vi "SRV_Sensor Config GUI.vi"(8 "error in (no error)":errorcluster, 9 "Sensor to Edit":string, 11 "Sensors Config File Path in":path) -> (0 "error out":errorcluster, 1 "Cancelled?":bool, 3 "Sensor Config Filepath":path)   [LabVIEW 2009]
doc: "A Producer-Consumer two-loop state machine template. This template uses the LPD Command Queues to drive its execution.\n\nThere are several advantages such as:\n- convenient error state control\n- the ability to pass data between states/loops/VIs via a variant\n- command history which is extremely valuable in troubleshooting when an error occurs\n\n\nAuthor: Mike Schultz\n\nLogicPD, Inc\nwww.logicpd.com"
uses:
  SRV_Sensor Config Cluster.ctl
  SRV_Sensor Analog-Digital.ctl
  SRV_Sensor Sampling Mode.ctl
  SRV_Sensor View Config Cluster.ctl
  SRV_Sensors Names.ctl
  SRV_Sensor PicoC Shared Var Type.ctl
  Support/SRV_Command-Data Queue Data Type.ctl
panel:
  in  "Sensor Config":T1={"Name"="", "A/D"=enum."Analog", "I2C Address"=0, "Register"=0, "Channel"=0, "Digital Mask"=0, "Units"="", "Sampling Mode"=enum."Polled", "Sample Period (ms)"=1000, "Formula"="", "Sensor View Config"={"Sensor Name"=enum."Gauge 01", "Minimum"=0.0, "Maximum"=10.0}, "Active"=FALSE, "PicoC Shared Var Type"=enum."Integer", "Index"=0, "Stream Multiple?"=FALSE, "Index End"=255} caption="Gauge 01" {"Register" format="%.0x"; "I2C Address" format="%.0x"; "Sample Period (ms)" min=10 max=60000 step=1; "Digital Mask" format="%.0x"; "Channel" format="%.0x"}
  in  "Cancel Button":bool
  in  "OK Button":bool
  in  "About":bool
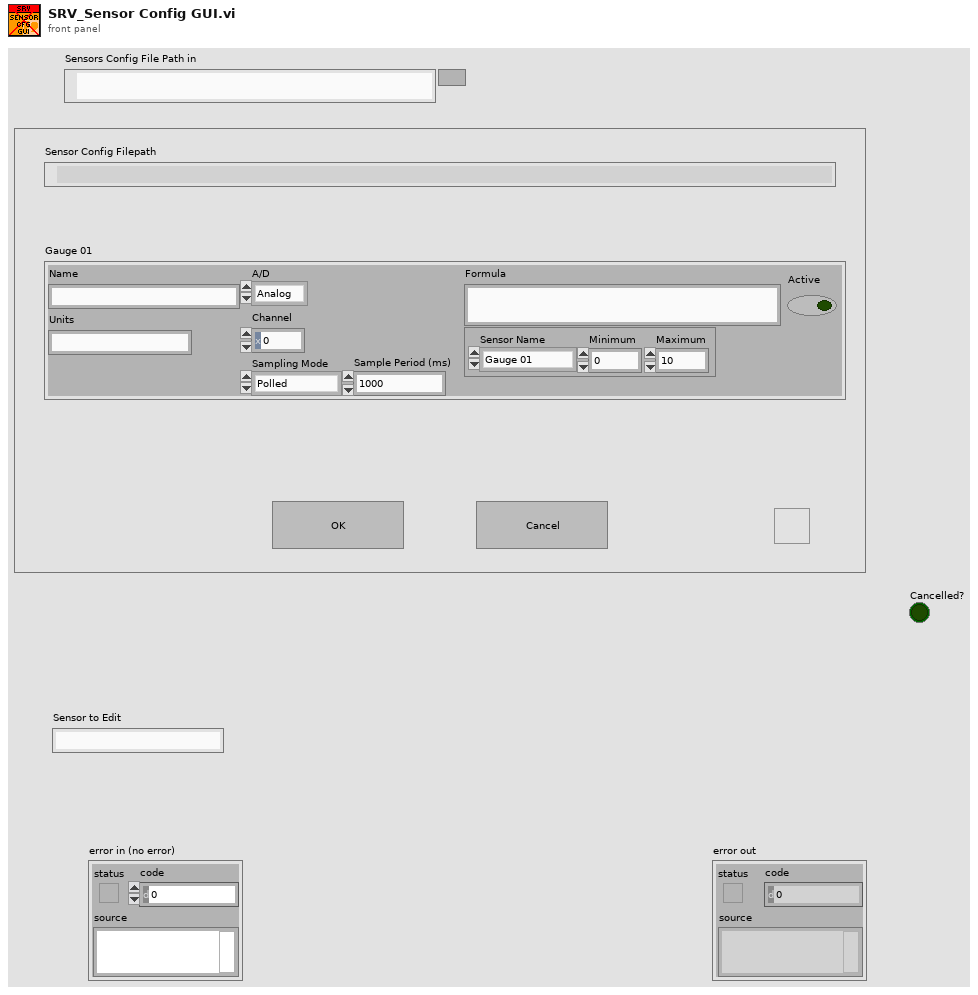
[diagram p1: front panel]
types:
  T1 = typedef "SRV_Sensor Config Cluster.ctl" = cluster{"Name":string, "A/D":T2, "I2C Address":u8, "Register":u8, "Channel":u8, "Digital Mask":u8, "Units":string, "Sampling Mode":T3, "Sample Period (ms)":u32, "Formula":string, "Sensor View Config":T4, "Active":bool, "PicoC Shared Var Type":T6, "Index":u8, "Stream Multiple?":bool, "Index End":u8}
  T2 = typedef "SRV_Sensor Analog-Digital.ctl" = enum16{"Analog", "Digital", "RCMx1 Analog", "PicoC Shared"}
  T3 = typedef "SRV_Sensor Sampling Mode.ctl" = enum16{"Polled", "Streaming"}
  T4 = typedef "SRV_Sensor View Config Cluster.ctl" = cluster{"Sensor Name":T5, "Minimum":dbl, "Maximum":dbl}
  T5 = typedef "SRV_Sensors Names.ctl" = enum16{"Gauge 01", "Gauge 02", "Gauge 03", "Gauge 04", "Meter 01", "Meter 02", "Meter 03", "Meter 04", "Numeric 01", "Numeric 02", "Numeric 03", "Numeric 04", "Numeric 05", "Numeric 06", "Numeric 07", "Numeric 08", "Boolean 01", "Boolean 02", "Boolean 03", "Boolean 04", "Boolean 05", "Boolean 06", "Boolean 07", "Boolean 08", "Boolean 09", "Boolean 10", "Boolean 11", "Boolean 12", "Boolean 13", "Boolean 14", "Boolean 15", "Boolean 16", "Boolean 17", "Boolean 18", "Boolean 19", "Boolean 20", "Boolean 21", "Boolean 22", "Boolean 23", "Boolean 24", "Boolean 25", "Boolean 26", "Boolean 27", "Boolean 28", "Boolean 29", "Boolean 30", "Boolean 31", "Boolean 32"}
  T6 = typedef "SRV_Sensor PicoC Shared Var Type.ctl" = enum16{"String", "Integer", "Float"}
  T7 = typedef "SRV_Command-Data Queue Data Type.ctl" = cluster{"Command":string, "Data":variant}
  T8 = cluster{"user event":refnum<user-event>, "Sensor Config Filepath":path, "Sensors Config":T1[], "Cancelled?":bool, "Sensor to Edit":T5, "Sensor Index":i32}
  T9 = enum8{"Enabled", "Disabled", "Disabled and Grayed Out"}
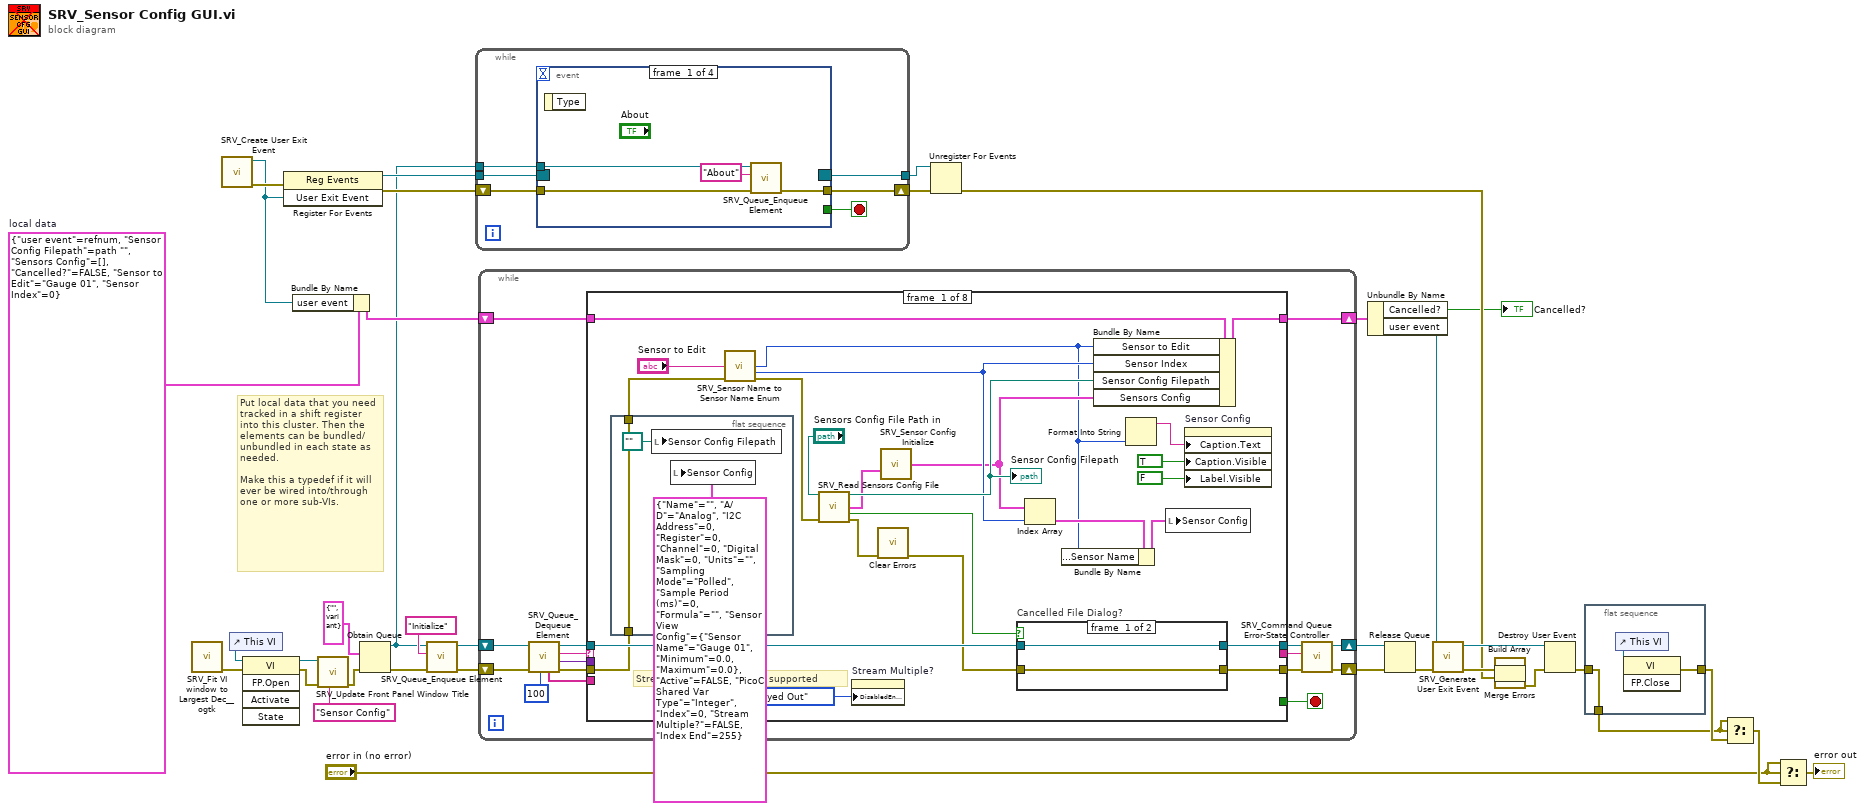
[diagram p0: block diagram]
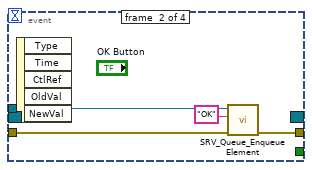
[diagram p2: hidden frame]
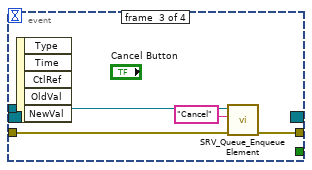
[diagram p3: hidden frame]
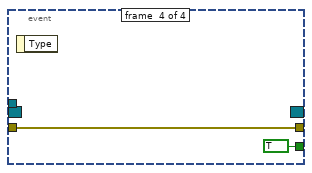
[diagram p4: hidden frame]
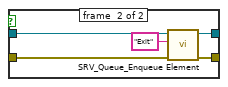
[diagram p5: hidden frame]
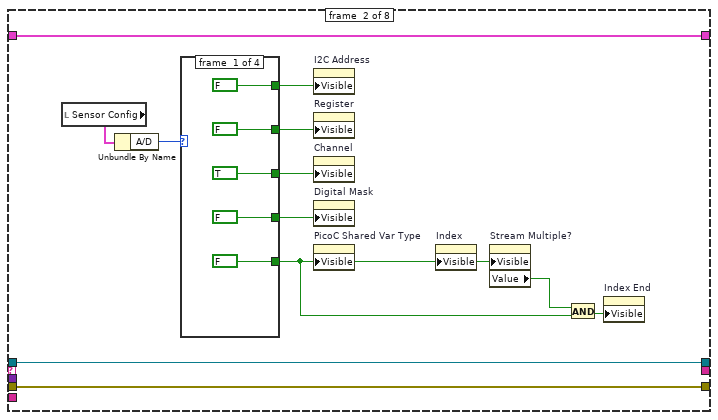
[diagram p6: hidden frame]
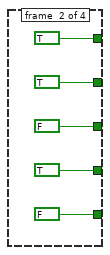
[diagram p7: hidden frame]
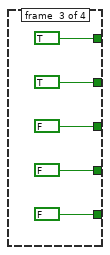
[diagram p8: hidden frame]
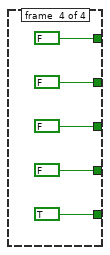
[diagram p9: hidden frame]
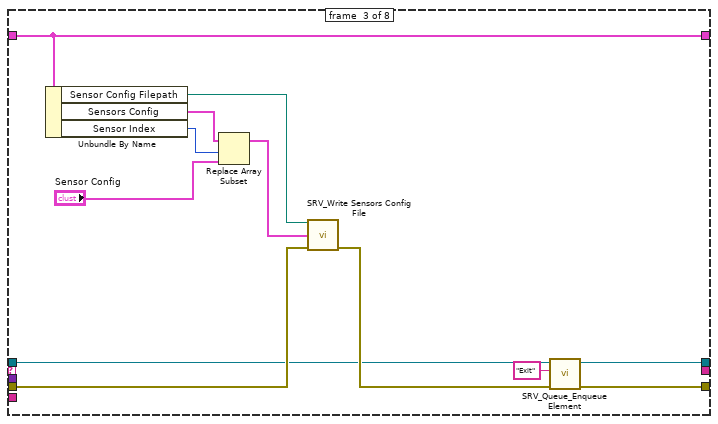
[diagram p10: hidden frame]
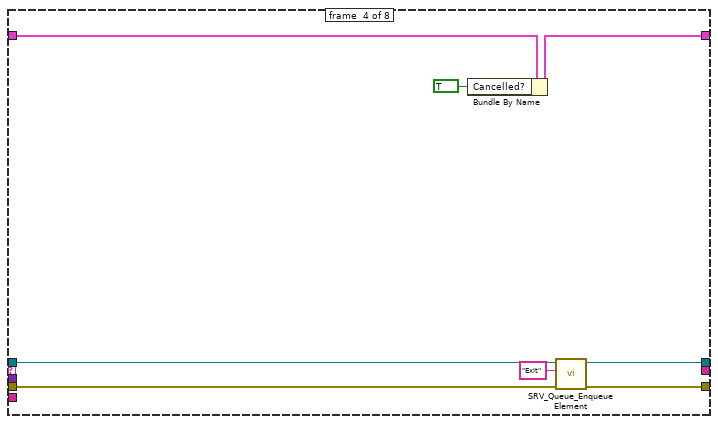
[diagram p11: hidden frame]
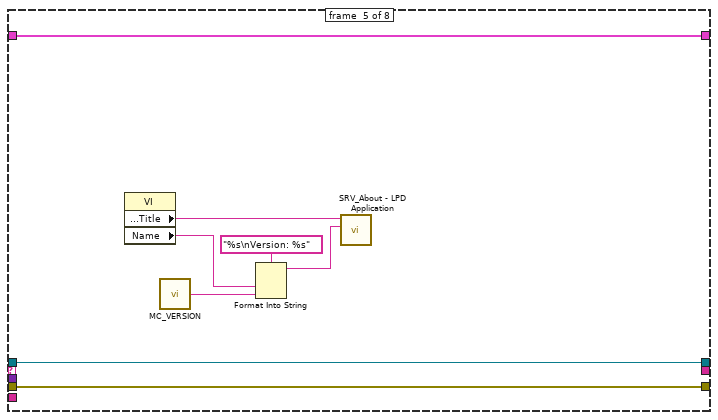
[diagram p12: hidden frame]
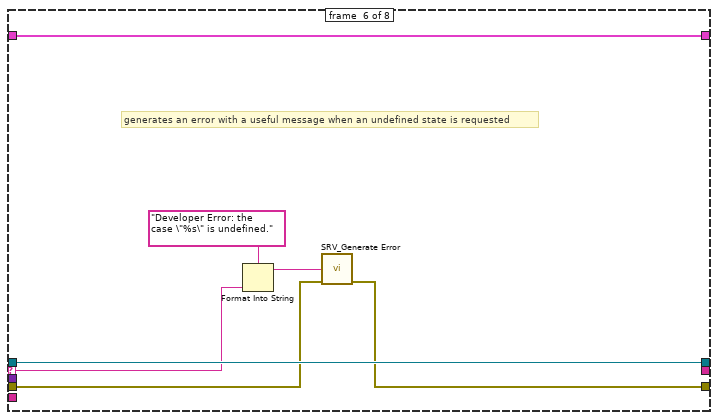
[diagram p13: hidden frame]
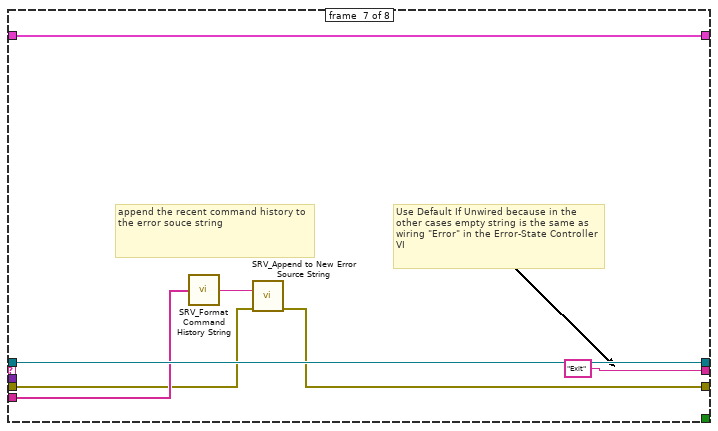
[diagram p14: hidden frame]
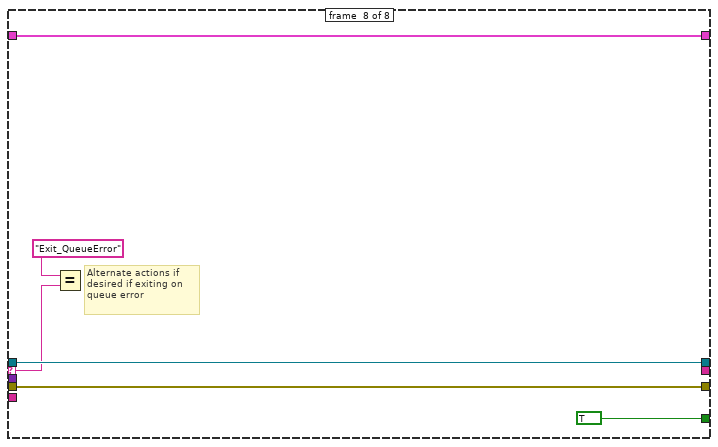
[diagram p15: hidden frame]
diagram:
  w31 = T8 {"user event"=refnum, "Sensor Config Filepath"=path "", "Sensors Config"=[], "Cancelled?"=FALSE, "Sensor to Edit"=enum."Gauge 01", "Sensor Index"=0}  # local data
  # "Put local data that you need tracked in a shift register into this cluster. Then the elements can be bundled/unbundled in each state as needed.\n\nMake this a typedef if it will ever be wired into/through one or more sub-VIs."
  n1 = call "SRV_Fit VI window to Largest Dec__ogtk.vi"() -> ("error out"=w9:errorcluster)  [unwired: 6 in, 1 out]
  n2 = call "SRV_Create User Exit Event.vi"() -> ("error out"=w22:errorcluster, "User Exit Event"=w21:refnum<user-event>)  [unwired: 10 in]
  n3 = control-ref of="This VI"() -> (w10:refnum<vi>)
  n4 = invoke class="VI" method="FP.Open"(reference=w10, error in=w9) -> (reference out=w6:refnum<vi>, error out=w5:errorcluster)  [unwired: 3 in, 3 out]
  n5 = register-events(error in=w22, w21) -> (reference out=w37:refnum<event-registration>, error out=w36:errorcluster)  [unwired: 1 in]
  n6 = Bundle By Name(cluster=w31, "user event"=w21) -> (w30:T8)
  n7 = call "SRV_Update Front Panel Window Title.vi"("Window Title Override String"="Sensor Config", "error in (no error)"=w5, "VI ref"=w6) -> ("error out"=w4:errorcluster)  [unwired: 7 in, 1 out]
  n8 = Obtain Queue(element data type=T7 {"Command"="", "Data"=variant} ("Queue Data Type"), error in (no error)=w4) -> (queue out=w17:refnum<queue>, error out=w18:errorcluster)  [unwired: 3 in, 1 out]
  n9 = call "SRV_Queue_Enqueue Element.vi"("error in (no error)"=w18, "Command"="Initialize", "Command-Data Queue"=w17) -> ("error out"=w14:errorcluster, "Command-Data Queue out"=w16:refnum<queue>)  [unwired: 6 in, 1 out]
  n10 = while {
    shift-right: [w42] -> w34
    shift-left: w36 -> [w43]
    tunnel: w17 -> [w41]
    tunnel: w37 -> [w40]
    tunnel: [w39] -> w35
    stop <- w38 stop-if-true
    n11 = event shown="[2] \"Cancel Button\": Value Change" {
      selector: w40 -> [_ _ _ _]
      dyn-events: [_ _ _ _] -> w39
      timeout: _ -> [_ _ _ _]
      tunnel: w43 -> [w47 w49 w53 w57]
      tunnel: [w46 w50 w54 w57] -> w42
      tunnel: w41 -> [w44 w48 w52 _]
      tunnel: [_ _ _ TRUE] -> w38
      event #0 {
        n12 = event-data() -> ()  [unwired: 1 in, 1 out]
        n13 = call "SRV_Queue_Enqueue Element.vi"("error in (no error)"=w47, "Command"="About", "Command-Data Queue"=w44) -> ("error out"=w46:errorcluster)  [unwired: 6 in, 2 out]
      }
      event #1 {
        n14 = event-data() -> ()  [unwired: 1 in, 5 out]
        n15 = call "SRV_Queue_Enqueue Element.vi"("error in (no error)"=w49, "Command"="OK", "Command-Data Queue"=w48) -> ("error out"=w50:errorcluster)  [unwired: 6 in, 2 out]
      }
      event #2 {
        n16 = event-data() -> ()  [unwired: 1 in, 5 out]
        n17 = call "SRV_Queue_Enqueue Element.vi"("error in (no error)"=w53, "Command"="Cancel", "Command-Data Queue"=w52) -> ("error out"=w54:errorcluster)  [unwired: 6 in, 2 out]
      }
      event #3 {
        n18 = event-data() -> ()  [unwired: 1 in, 1 out]
      }
    }
  }
  n19 = while {
    shift-right: [w67] -> w33
    shift-left: w14 -> [w73]
    shift-right: [w65] -> w32
    shift-left: w16 -> [w71]
    shift-right: [w59] -> w29
    shift-left: w30 -> [w60]
    stop <- w61 stop-if-true
    n20 = call "SRV_Queue_Dequeue Element.vi"("timeout in ms (-1)"=100, "error in (no error)"=w73, "Command-Data Queue"=w71) -> ("error out"=w72:errorcluster, "Data"=w64:variant, "Command"=w69:string, "Command-Data Queue out"=w70:refnum<queue>, "Command History"=w63:string[])  [unwired: 3 in, 1 out]
    n21 = case shown="\"About\"" w69 {
      selector: w69 -> [_ _ _ _ _ w172 _ w184]
      tunnel: w72 -> [w91 w118 w149 w158 w166 w170 w176 w186]
      tunnel: [w95 w118 w146 w157 w166 w169 w177 w186] -> w68
      tunnel: w70 -> [w96 w119 w145 w159 w167 w174 w181 w187]
      tunnel: [w94 w119 w144 w156 w167 w174 w181 w187] -> w66
      tunnel: w64 -> [_ _ _ _ _ _ _ _]
      tunnel: w63 -> [_ _ _ _ _ _ w180 _]
      tunnel: [_ _ _ _ _ _ "Exit" ("Error Command") _] -> w62
      tunnel: [_ _ _ _ _ _ _ TRUE] -> w61
      tunnel: w60 -> [w78 w116 w151 w154 w161 w171 w178 w182]
      tunnel: [w93 w116 w151 w153 w161 w171 w178 w182] -> w59
      frame #0 {
        # "Streaming multiple not yet supported"
        n22 = flat-sequence {
          tunnel: w91 -> [w99]
          tunnel: [w99] -> w88
          frame #0 {
            n23 = local write "Sensor Config Filepath"(path "" ("Sensor Config Filepath")) -> ()
            n24 = local write "Sensor Config"(T1 {"Name"="", "A/D"=enum."Analog", "I2C Address"=0, "Register"=0, "Channel"=0, "Digital Mask"=0, "Units"="", "Sampling Mode"=enum."Polled", "Sample Period (ms)"=0, "Formula"="", "Sensor View Config"={"Sensor Name"=enum."Gauge 01", "Minimum"=0.0, "Maximum"=0.0}, "Active"=FALSE, "PicoC Shared Var Type"=enum."Integer", "Index"=0, "Stream Multiple?"=FALSE, "Index End"=255} ("Sensor Config")) -> ()
          }
        }
        n25 = call "SRV_Sensor Name to Sensor Name Enum.vi"("Sensor to Edit"="Sensor to Edit", "error in (no error)"=w88) -> ("Sensor View Indicator Names"=w81:T5, "Sensor Index"=w86:i32, "error out"=w87:errorcluster)  [unwired: 11 in]
        n26 = call "SRV_Read Sensors Config File.vi"("Sensors Config File Path"="Sensors Config File Path in", "error in (no error)"=w87) -> ("Sensors Config File Path out"=w92:path, "Sensors Config"=w85:T1[], "Cancelled?"=w97:bool, "error out"=w80:errorcluster)  [unwired: 10 in]
        "Sensor Config Filepath" <- w92
        n27 = property on="Stream Multiple?" class="Bool (strict)"("DisabledEnum"=T9."Disabled and Grayed Out" ("Disabled")) -> ()  [unwired: 2 in, 2 out]
        n28 = call <vilib>:"Clear Errors.vi"("error in (no error)"=w80) -> ("error out"=w79:errorcluster)  [unwired: 6 in]
        n29 = call "SRV_Sensor Config Initialize.vi"("Sensors Config"=w85) -> ("Sensors Config out"=w84:T1[])  [unwired: 13 in, 1 out]
        n30 = case "Cancelled File Dialog?" shown="True" w97 {
          tunnel: w79 -> [w101 w106]
          tunnel: w96 -> [w102 w107]
          tunnel: [w101 w105] -> w95
          tunnel: [w102 w104] -> w94
          frame #0 {
          }
          frame #1 {
            n31 = call "SRV_Queue_Enqueue Element.vi"("error in (no error)"=w106, "Command"="Exit", "Command-Data Queue"=w107) -> ("error out"=w105:errorcluster, "Command-Data Queue out"=w104:refnum<queue>)  [unwired: 6 in, 1 out]
          }
        }
        n32 = Index Array(array=w84, index=w86) -> (element=w83:T1)
        n33 = Bundle By Name(cluster=w83, "Sensor View Config.Sensor Name"=w81) -> (w82:T1)
        n34 = Bundle By Name(cluster=w78, "Sensor to Edit"=w81, "Sensor Index"=w86, "Sensor Config Filepath"=w92, "Sensors Config"=w84) -> (w93:T8)
        n35 = Format Into String(w81) -> (resulting string=w75:string)  [unwired: 3 in, 1 out]
        n36 = local write "Sensor Config"(w82) -> ()
        n37 = property on="Sensor Config" class="Clust (strict)"("Caption.Text"=w75, "Caption.Visible"=TRUE, "Label.Visible"=FALSE) -> ()  [unwired: 2 in, 2 out]
      }
      frame #1 {
        n38 = local read "Sensor Config"() -> (w117:T1)
        n39 = Unbundle By Name(w117) -> ("A/D"=w115:T2)
        n40 = case shown="\"RCMx1 Analog\"" w115 {
          tunnel: [FALSE ("Visible") TRUE ("Visible") TRUE ("Visible") FALSE ("Visible")] -> w114
          tunnel: [FALSE ("Visible") TRUE ("Visible") TRUE ("Visible") FALSE ("Visible")] -> w113
          tunnel: [TRUE ("Visible") FALSE ("Visible") FALSE ("Visible") FALSE ("Visible")] -> w112
          tunnel: [FALSE ("Visible") TRUE ("Visible") FALSE ("Visible") FALSE ("Visible")] -> w111
          tunnel: [FALSE ("Visible") FALSE ("Visible") FALSE ("Visible") TRUE ("Visible")] -> w109
          frame #0 {
          }
          frame #1 {
          }
          frame #2 {
          }
          frame #3 {
          }
        }
        n41 = property on="I2C Address" class="DigNum (strict)"("Visible"=w114) -> ()  [unwired: 2 in, 2 out]
        n42 = property on="Register" class="DigNum (strict)"("Visible"=w113) -> ()  [unwired: 2 in, 2 out]
        n43 = property on="Channel" class="DigNum (strict)"("Visible"=w112) -> ()  [unwired: 2 in, 2 out]
        n44 = property on="Digital Mask" class="DigNum (strict)"("Visible"=w111) -> ()  [unwired: 2 in, 2 out]
        n45 = property on="PicoC Shared Var Type" class="Enum (strict)"("Visible"=w109) -> ()  [unwired: 2 in, 2 out]
        n46 = property on="Index" class="DigNum (strict)"("Visible"=w109) -> ()  [unwired: 2 in, 2 out]
        n47 = property on="Stream Multiple?" class="Bool (strict)"("Visible"=w109) -> ("Value"=w108:bool)  [unwired: 2 in, 2 out]
        n48 = And(x=w108, y=w109) -> (x .and. y?=w110:bool)
        n49 = property on="Index End" class="DigNum (strict)"("Visible"=w110) -> ()  [unwired: 2 in, 2 out]
      }
      frame #2 {
        n50 = Unbundle By Name(w151) -> ("Sensor Config Filepath"=w150:path, "Sensors Config"=w143:T1[], "Sensor Index"=w141:i32)
        n51 = Replace Array Subset(array=w143, new element="Sensor Config", index=w141) -> (w142:T1[])
        n52 = call "SRV_Write Sensors Config File.vi"("Sensors Config File Path"=w150, "Sensors Config"=w142, "error in (no error)"=w149) -> ("error out"=w147:errorcluster)  [unwired: 12 in]
        n53 = call "SRV_Queue_Enqueue Element.vi"("error in (no error)"=w147, "Command"="Exit", "Command-Data Queue"=w145) -> ("error out"=w146:errorcluster, "Command-Data Queue out"=w144:refnum<queue>)  [unwired: 6 in, 1 out]
      }
      frame #3 {
        n54 = Bundle By Name(cluster=w154, "Cancelled?"=TRUE) -> (w153:T8)
        n55 = call "SRV_Queue_Enqueue Element.vi"("error in (no error)"=w158, "Command"="Exit", "Command-Data Queue"=w159) -> ("error out"=w157:errorcluster, "Command-Data Queue out"=w156:refnum<queue>)  [unwired: 6 in, 1 out]
      }
      frame #4 {
        n56 = property class="VI"() -> ("Front Panel.Title"=w165:string, "Name"=w162:string)  [unwired: 2 in, 2 out]
        n57 = call "MC_VERSION.vi"() -> ("MC Version"=w160:string)
        n58 = Format Into String(format string="%s\nVersion: %s", w162, w160) -> (resulting string=w163:string)  [unwired: 2 in, 1 out]
        n59 = call "SRV_About - LPD Application.vi"("Version Info"=w163, "Application Name"=w165) -> ()  [unwired: 10 in]
      }
      frame #5 {
        # "generates an error with a useful message when an undefined state is requested"
        n60 = Format Into String(format string="Developer Error: the case \"%s\" is undefined.", w172) -> (resulting string=w168:string)  [unwired: 2 in, 1 out]
        n61 = call "SRV_Generate Error.vi"("Message"=w168, "error in (no error)"=w170) -> ("error out"=w169:errorcluster)  [unwired: 13 in]
      }
      frame #6 {
        # "Use Default If Unwired because in the other cases empty string is the same as wiring \"Error\" in the Error-State Controller VI"
        # "append the recent command history to the error souce string"
        n62 = call "SRV_Format Command History String.vi"("Command History"=w180) -> ("Command History String"=w175:string)  [unwired: 14 in]
        n63 = call "SRV_Append to New Error Source String.vi"("Message String to append"=w175, "Error In (no error)"=w176) -> ("error out"=w177:errorcluster)  [unwired: 13 in]
      }
      frame #7 {
        # "Alternate actions if desired if exiting on queue error"
        n64 = Equal?(x="Exit_QueueError", y=w184) -> ()  [unwired: 1 out]
      }
    }
    n65 = call "SRV_Command Queue Error-State Controller.vi"("error in (no error)"=w68, "Error Command"=w62, "Command-Data Queue"=w66) -> ("error out"=w67:errorcluster, "Command-Data Queue out"=w65:refnum<queue>)  [unwired: 7 in]
  }
  n66 = Unregister For Events(event registration refnum=w35, error in=w34) -> (error out=w24:errorcluster)
  n67 = Unbundle By Name(w29) -> ("Cancelled?"=→"Cancelled?":bool, "user event"=w28:refnum<user-event>)
  n68 = Release Queue(queue=w32, error in (no error)=w33) -> (error out=w27:errorcluster)  [unwired: 1 in, 2 out]
  n69 = call "SRV_Generate User Exit Event.vi"("error in (no error)"=w27, "User Exit Event"=w28) -> ("error out"=w25:errorcluster, "User Exit Event out"=w26:refnum<user-event>)  [unwired: 8 in]
  n70 = Build Array(w25, w24) -> (w20:errorcluster[])
  n71 = call <vilib>:"Merge Errors.vi"("error array in"=w20) -> ("error out"=w23:errorcluster)  [unwired: 6 in]
  n72 = Destroy User Event(user event=w26, error in=w23) -> (error out=w12:errorcluster)
  n73 = flat-sequence {
    tunnel: [w190] -> w13
    tunnel: w12 -> [w189]
    tunnel: [w189] -> w11
    frame #0 {
      n74 = control-ref of="This VI"() -> (w188:refnum<vi>)
      n75 = invoke class="VI" method="FP.Close"(reference=w188) -> (error out=w190:errorcluster)  [unwired: 2 in, 2 out]
    }
  }
  n76 = Select(t=w11, s=w11, f=w13) -> (s? t:f=w2:errorcluster)
  n77 = Select(t="error in (no error)", s="error in (no error)", f=w2) -> (s? t:f=→"error out":errorcluster)
